vi "Display Confirmation to User.vi"(6 "Calling VI in":refnum<vi>, 7 "Confirmation Type":T5, 8 "error in (no error)":errorcluster, 11 "Config":T1) -> (0 "error out":errorcluster, 1 "New Config?":bool, 2 "OK?":bool, 3 "Config out":T1)   [LabVIEW 2023, in "VI Properties Editor.lvlib"]
doc: "Displays a confirmation dialog to the user, taking into account <B>Confirmation Type</B> and <B>Config</B>."
uses:
  VI Properties Editor.lvlib
  CTLs/Confirmation Type.ctl
  CTLs/Config.ctl
  CTLs/Column Name.ctl
  CTLs/Filter Type.ctl
  CTLs/Filter Info.ctl
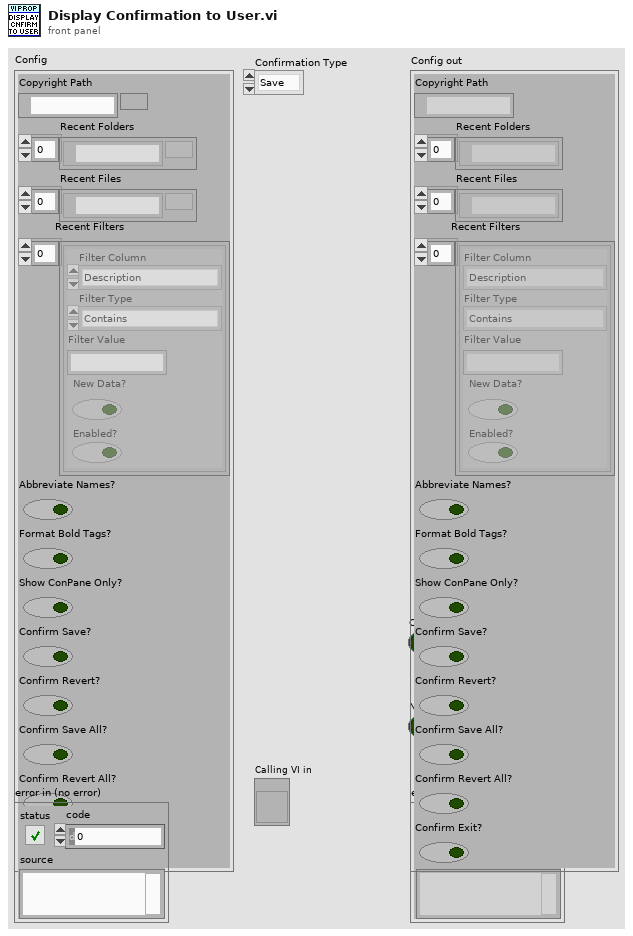
[diagram p1: front panel]
types:
  T1 = typedef "VI Properties Editor.lvlib/Config.ctl" = cluster{"Copyright Path":path, "Recent Folders":path[], "Recent Files":path[], "Recent Filters":T2[], "Abbreviate Names?":bool, "Format Bold Tags?":bool, "Show ConPane Only?":bool, "Confirm Save?":bool, "Confirm Revert?":bool, "Confirm Save All?":bool, "Confirm Revert All?":bool, "Confirm Exit?":bool}
  T2 = typedef "VI Properties Editor.lvlib/Filter Info.ctl" = cluster{"Filter Column":T3, "Filter Type":T4, "Filter Value":string, "New Data?":bool, "Enabled?":bool}
  T3 = typedef "VI Properties Editor.lvlib/Column Name.ctl" = enum16{"Name", "Path", "Type", "Window Title", "Description", "Help Path", "Help Tag", "Custom Title?", "Reentrant?", "Inlined?"}
  T4 = typedef "VI Properties Editor.lvlib/Filter Type.ctl" = enum16{"Contains", "Equals", "Starts with", "Ends with", "Does not contain", "Does not equal", "Is empty", "Is not empty"}
  T5 = typedef "VI Properties Editor.lvlib/Confirmation Type.ctl" = enum16{"Save", "Revert", "Save All", "Revert All"}
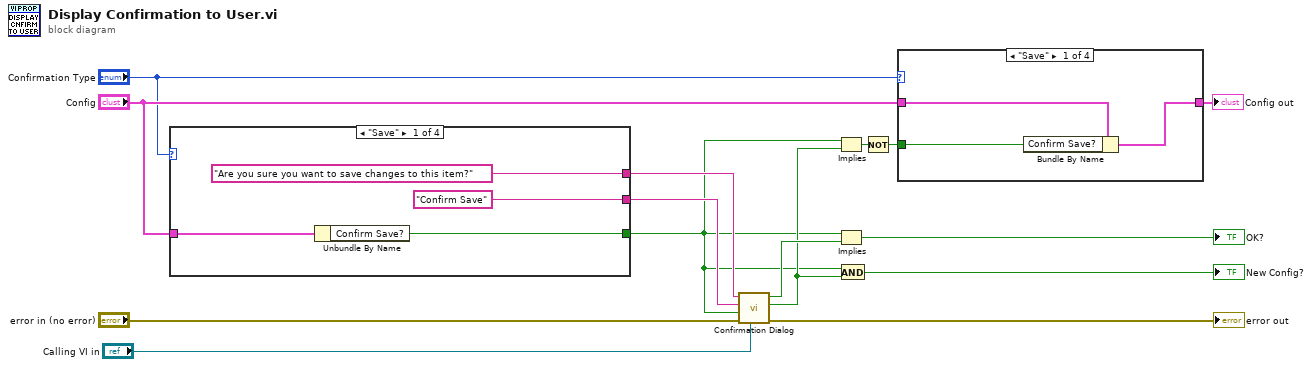
[diagram p0: block diagram]
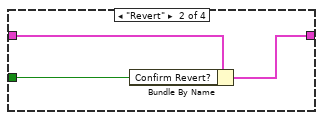
[diagram p2: hidden frame]
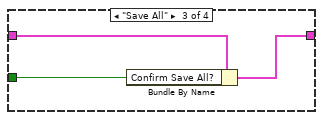
[diagram p3: hidden frame]
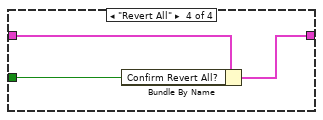
[diagram p4: hidden frame]
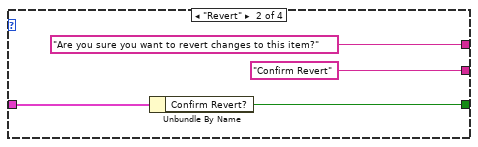
[diagram p5: hidden frame]
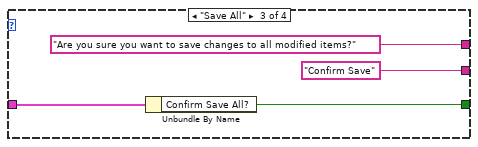
[diagram p6: hidden frame]
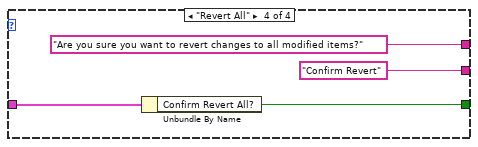
[diagram p7: hidden frame]
diagram:
  n1 = case shown="\"Save\"" "Confirmation Type" {
    tunnel: ["Are you sure you want to save changes to this item?" "Are you sure you want to revert changes to this item?" "Are you sure you want to save changes to all modified items?" "Are you sure you want to revert changes to all modified items?"] -> w12
    tunnel: "Config" -> [w18 w22 w26 w30]
    tunnel: [w17 w21 w25 w29] -> w3
    tunnel: ["Confirm Save" "Confirm Revert" "Confirm Save" "Confirm Revert"] -> w15
    frame "Save" {
      n2 = Unbundle By Name(w18) -> ("Confirm Save?"=w17:bool)
    }
    frame "Revert" {
      n3 = Unbundle By Name(w22) -> ("Confirm Revert?"=w21:bool)
    }
    frame "Save All" {
      n4 = Unbundle By Name(w26) -> ("Confirm Save All?"=w25:bool)
    }
    frame "Revert All" {
      n5 = Unbundle By Name(w30) -> ("Confirm Revert All?"=w29:bool)
    }
  }
  n6 = call "Confirmation Dialog.vi"("Calling VI in"="Calling VI in", "error in (no error)"="error in (no error)", "Enable"=w3, "Window Title (\"\")"=w15, "Message"=w12) -> ("error out"=→"error out":errorcluster, "Skip Prompts?"=w5:bool, "OK?"=w6:bool)  [unwired: 4 in]
  n7 = Implies(1:w5, 2:w3) -> (0:w8:bool)
  n8 = Implies(1:w6, 2:w3) -> (0:→"OK?":bool)
  n9 = And(x=w3, y=w5) -> (x .and. y?=→"New Config?":bool)
  n10 = Not(x=w8) -> (.not. x?=w2:bool)
  n11 = case shown="\"Save\"" "Confirmation Type" {
    tunnel: "Config" -> [w34 w37 w40 w43]
    tunnel: [w33 w36 w39 w42] -> w7
    tunnel: w2 -> [w32 w35 w38 w41]
    frame "Save" {
      n12 = Bundle By Name(cluster=w34, "Confirm Save?"=w32) -> (w33:T1)
    }
    frame "Revert" {
      n13 = Bundle By Name(cluster=w37, "Confirm Revert?"=w35) -> (w36:T1)
    }
    frame "Save All" {
      n14 = Bundle By Name(cluster=w40, "Confirm Save All?"=w38) -> (w39:T1)
    }
    frame "Revert All" {
      n15 = Bundle By Name(cluster=w43, "Confirm Revert All?"=w41) -> (w42:T1)
    }
  }
  "Config out" <- w7
